vi "picoquant_shove_into_processing_queue.vi"(8 "error in (no error)":errorcluster, 10 "data_in":T1, 11 "picoquant_generic in":refnum<class "picoquant_generic.lvclass">) -> (0 "error out":errorcluster, 3 "picoquant_generic out":refnum<class "picoquant_generic.lvclass">)   [LabVIEW 2015, in "picoquant_generic.lvclass"]
uses:
  picoquant_generic.lvclass
  picoquant_data_tdef.ctl
  picoquant_generic.lvclass/picoquant_generic.ctl
  processing_tasks_tdef.ctl
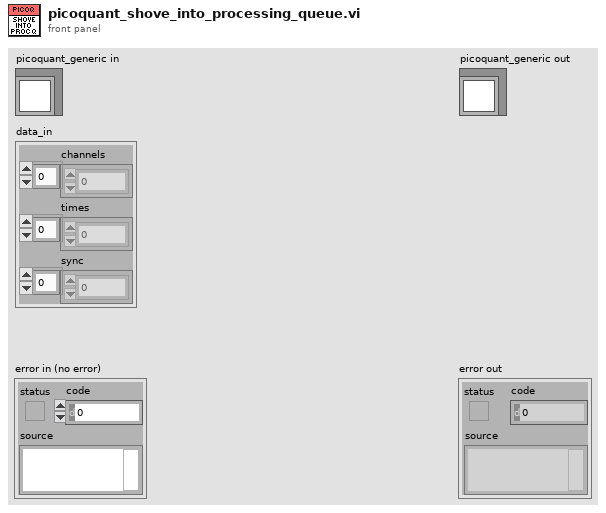
[diagram p1: front panel]
types:
  T1 = typedef "picoquant_data_tdef.ctl" = cluster{"channels":u8[], "times":u64[], "sync":u64[]}
  T2 = typedef "processing_tasks_tdef.ctl" = enum16{"none", "correlate", "histogram"}
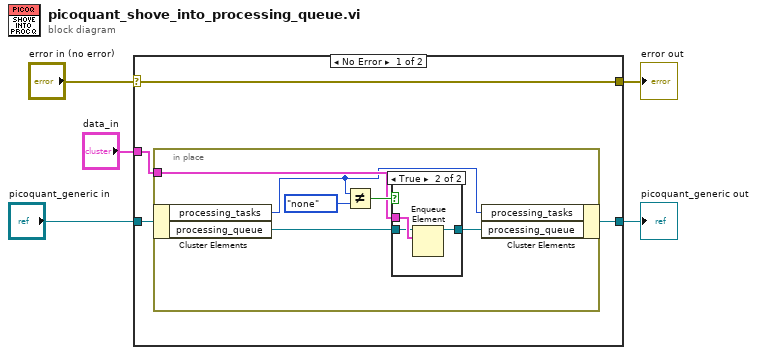
[diagram p0: block diagram]
diagram:
  n1 = case shown="No Error" "error in (no error)" {
    selector: "error in (no error)" -> [w9 w21]
    tunnel: [w9 w21] -> w4
    tunnel: [w6 w20] -> w2
    tunnel: "picoquant_generic in" -> [w7 w20]
    tunnel: "data_in" -> [w8 _]
    frame No Error {
      n2 = in-place {
        in-place-border: w8 -> [w13]
        n3 = in-place-cluster #1(w7) -> ("processing_tasks"=w10:T2, "processing_queue"=w12:refnum<queue>)
        n4 = Not Equal?(x=w10, y=processing_tasks_tdef."none") -> (x != y?=w14:bool)
        n5 = case shown="True" w14 {
          tunnel: w13 -> [_ w19]
          tunnel: w12 -> [w16 w18]
          tunnel: [w16 w17] -> w11
          frame False {
          }
          frame True {
            n6 = Enqueue Element(queue=w18, element=w19) -> (queue out=w17:refnum<queue>)  [unwired: 2 in, 2 out]
          }
        }
        n7 = in-place-cluster #1("processing_tasks"=w10, "processing_queue"=w11) -> (w6:refnum<class "picoquant_generic.lvclass">)
      }
    }
    frame Error {
    }
  }
  "error out" <- w4
  "picoquant_generic out" <- w2
